vi "Node - Config Reader.vi"(8 "error in (no error)":errorcluster, 11 "Node Data In":T1) -> (0 "error out":errorcluster, 3 "Node Data Out":T1)   [LabVIEW 2016, in "PXImc Router.lvlib"]
uses:
  PXImc Router.lvlib
  Controls/Node Data.ctl
  <vilib>/NI Veristand/VeriStand Data/Byte Buffer/Byte Buffer.lvclass
  Controls/Node/Node - PXImc Parameters.ctl
  Controls/Node/Transfer Data.ctl
  Controls/Node/Node Ch Properties.ctl
  Controls/Data Type.ctl
  <vilib>/NI Veristand/VeriStand Data/Byte Buffer/Byte Buffer.lvclass/Byte Buffer.ctl
  <vilib>/NI Veristand/VeriStand Data/Byte Buffer/Byte Buffer.Get Buffer Pointer.vi
  <vilib>/NI Veristand/VeriStand Data/Byte Buffer/Byte Buffer.Get Buffer Size.vi
  <vilib>/NI Veristand/VeriStand Data/Memory Management/Memory Management.MoveByteBlock (Pointer).vi
  <vilib>/NI Veristand/VeriStand Data/Pointer Operations/Pointer.New.vi
  <vilib>/NI Veristand/VeriStand Data/Pointer Operations/Pointer.Dispose.vi
  <vilib>/NI Veristand/VeriStand Data/Byte Buffer/Byte Buffer.Set Buffer Pointer.vi
  <vilib>/NI Veristand/VeriStand Data/Byte Buffer/Byte Buffer.Set Buffer Size.vi
  <vilib>/NI Veristand/VeriStand Data/Memory Management/Memory Management.Handle Return.vi
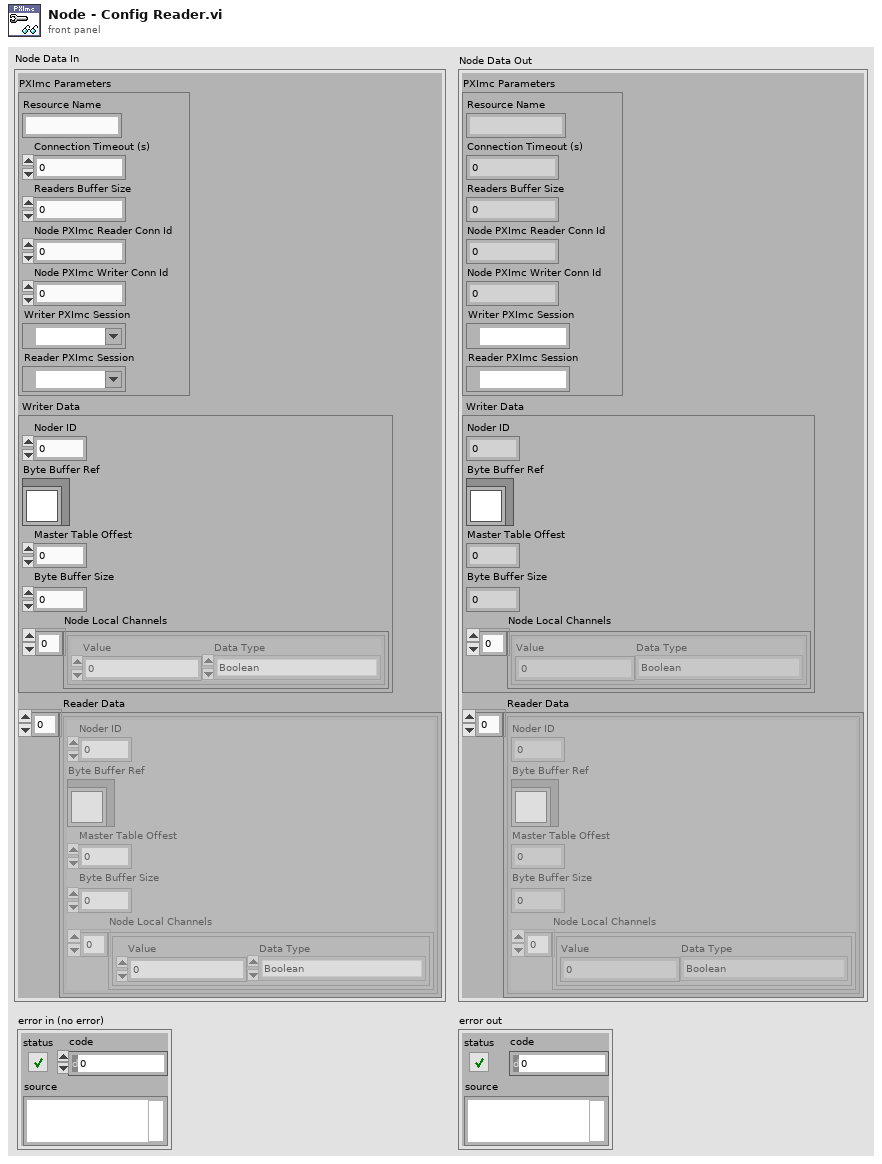
[diagram p1: front panel]
types:
  T1 = typedef "PXImc Router.lvlib/Node Data.ctl" = cluster{"PXImc Parameters":T2, "Writer Data":T3, "Reader Data":T3[]}
  T2 = typedef "PXImc Router.lvlib/Node - PXImc Parameters.ctl" = cluster{"Resource Name":string, "Connection Timeout (s)":dbl, "Readers Buffer Size":u32, "Node PXImc Reader Conn Id":u16, "Node PXImc Writer Conn Id":u16, "Writer PXImc Session":refnum<k21>, "Reader PXImc Session":refnum<k21>}
  T3 = typedef "PXImc Router.lvlib/Transfer Data.ctl" = cluster{"Noder ID":u32, "Byte Buffer Ref":refnum<class "Byte Buffer.lvclass">, "Master Table Offest":u32, "Byte Buffer Size":u32, "Node Local Channels":T4[]}
  T4 = typedef "PXImc Router.lvlib/Node Ch Properties.ctl" = cluster{"Value":dbl, "Data Type":T5}
  T5 = typedef "PXImc Router.lvlib/Data Type.ctl" = enum16{"Boolean", "SGL", "DBL", "I8", "I16", "I32", "I64", "U8", "U16", "U32", "U64"}
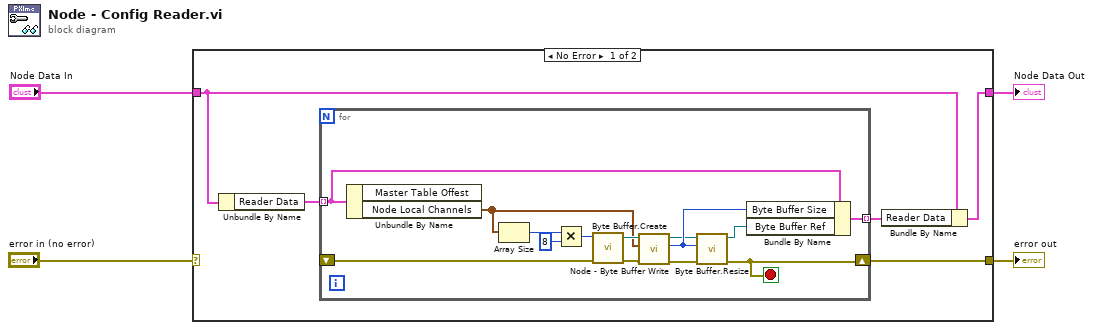
[diagram p0: block diagram]
diagram:
  n1 = case shown="No Error" "error in (no error)" {
    selector: "error in (no error)" -> [_ w25]
    tunnel: [w7 w24] -> w4
    tunnel: [w6 w25] -> w3
    tunnel: "Node Data In" -> [w5 w24]
    frame No Error {
      n2 = Unbundle By Name(w5) -> ("Reader Data"=w8:T3[])
      n3 = for {
        tunnel: w8 -> [w10] mode=indexing
        shift-right: [w17] -> w6
        shift-left: _ -> [w20]
        tunnel: [w18] -> w9 mode=indexing
        stop <- w17 stop-if-true
        n4 = Unbundle By Name(w10) -> ("Node Local Channels"=w11:T4[])  [unwired: 1 out]
        n5 = Array Size(array=w11) -> (size(s)=w23:i32)
        n6 = Multiply(x=w23, y=8) -> (x*y=w21:i32)
        n7 = call <vilib>:"Byte Buffer.Create.vi"("error in (no error)"=w20, "size"=w21) -> ("error out"=w12:errorcluster, "Byte Buffer"=w16:refnum<class "Byte Buffer.lvclass">)  [unwired: 8 in]
        n8 = call "Node - Byte Buffer Write.vi"("error in (no error)"=w12, "Node Local Channels"=w11, "Byte Buffer In"=w16) -> ("error out"=w13:errorcluster, "Buffer Offset Out"=w15:u64, "Byte Buffer Out"=w14:refnum<class "Byte Buffer.lvclass">)  [unwired: 6 in]
        n9 = call <vilib>:"Byte Buffer.Resize.vi"("error in (no error)"=w13, "new size"=w15, "Byte Buffer in"=w14) -> ("error out"=w17:errorcluster, "Byte Buffer out"=w19:refnum<class "Byte Buffer.lvclass">)  [unwired: 7 in]
        n10 = Bundle By Name(cluster=w10, "Byte Buffer Size"=w15, "Byte Buffer Ref"=w19) -> (w18:T3)
      }
      n11 = Bundle By Name(cluster=w5, "Reader Data"=w9) -> (w7:T1)
    }
    frame Error {
    }
  }
  "error out" <- w3
  "Node Data Out" <- w4
